vi "Close.vi"(8 "error in (no error)":errorcluster, 11 "VISA resource name":refnum<visa-resource-name>) -> (0 "error out":errorcluster)   [LabVIEW 2011, in "Yokogawa DX Series.lvlib"]
doc: "This VI closes the I/O interface with the instrument."
uses:
  <instrlib>/Yokogawa DX Series/Yokogawa DX Series.lvlib
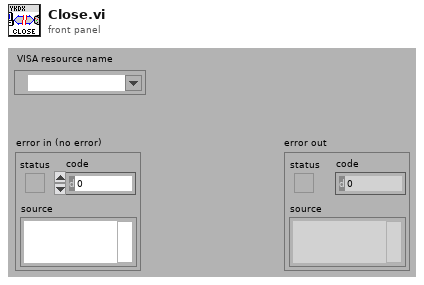
[diagram p1: front panel]
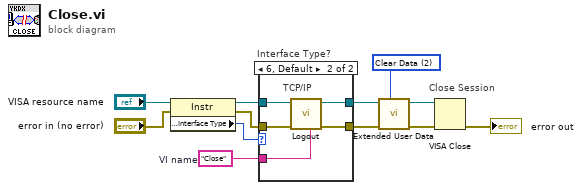
[diagram p0: block diagram]
diagram:
  w1 = 2 items=["Read Data", "Write Data", "Clear Data", "Clear All Data"] ("Action")
  w10 = "Close"  # VI name
  # "Close Session"
  n1 = property class="Instr"(reference="VISA resource name", error in="error in (no error)") -> (reference out=w7:refnum<visa-resource-name>, error out=w9:errorcluster, "Interface Information:Interface Type"=w6:u16)
  n2 = case "Interface Type?" shown="6, Default" w6 {
    tunnel: [w13 w19] -> w4
    tunnel: [w14 w18] -> w5
    tunnel: w10 -> [_ w15]
    tunnel: w9 -> [w13 w16]
    tunnel: w7 -> [w14 w17]
    frame 4 {
      # "Serial"
    }
    frame 6, Default {
      # "TCP/IP"
      n3 = call <instrlib>:"Logout.vi"("Source (\"\")"=w15, "error in (no error)"=w16, "VISA resource name"=w17) -> ("error out"=w19:errorcluster, "VISA resource name out"=w18:refnum<visa-resource-name>)  [unwired: 7 out]
    }
  }
  n4 = call <instrlib>:"Extended User Data.vi"("Action (0 : Read Data)"=w1, "error in (no error)"=w4, "VISA resource name"=w5) -> ("error out"=w2:errorcluster, "VISA resource name out"=w3:refnum<visa-resource-name>)  [unwired: 1 in, 6 out]
  n5 = VISA Close(VISA resource name=w3, error in (no error)=w2) -> (error out=→"error out":errorcluster)
